vi "ConstructLabVIEWItem.vi"(8 "error in (no error)":errorcluster, 9 "Path":path, 10 "Qualified name":string, 11 "CLabVIEWItem in":refnum<class "CLabVIEWItem.lvclass">) -> (0 "error out":errorcluster, 3 "CLabVIEWItem out":refnum<class "CLabVIEWItem.lvclass">)   [LabVIEW 2020, in "LabVIEWItem.lvlib" / "CLabVIEWItem.lvclass"]
uses:
  CLabVIEWItem.lvclass
  CLabVIEWItem.lvclass/CLabVIEWItem.ctl
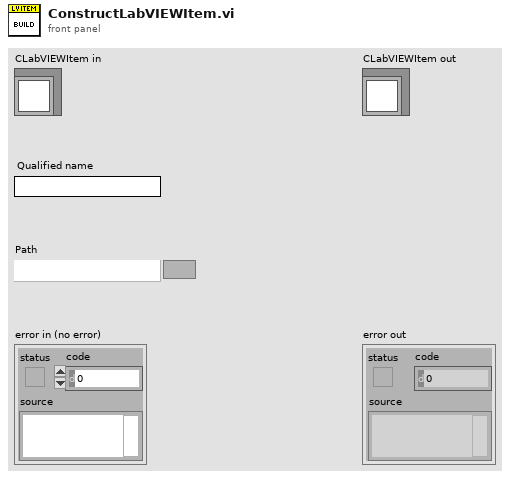
[diagram p1: front panel]
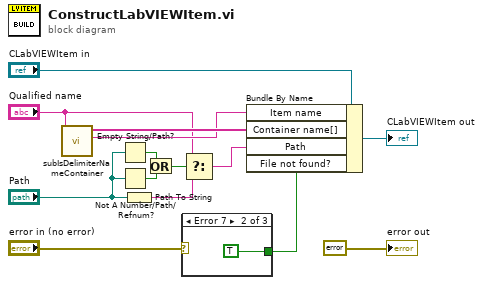
[diagram p0: block diagram]
diagram:
  n1 = call "subIsDelimiterNameContainer.vi"("delimited name"="Qualified name") -> ("item name"=w2:string, "container name[]"=w14:string[])  [unwired: 8 in, 1 out]
  n2 = Empty String/Path?(string/path="Path") -> (empty?=w12:bool)
  n3 = Not A Number/Path/Refnum?(number/path/refnum="Path") -> (NaN/Path/Refnum?=w11:bool)
  n4 = Path To String(path="Path") -> (string=w9:string)
  n5 = Or(x=w12, y=w11) -> (x .or. y?=w10:bool)
  n6 = case shown="Error 7" "error in (no error)" {
    tunnel: [_ TRUE _] -> w6
    frame No Error {
    }
    frame Error {
    }
    frame Default {
    }
  }
  n7 = Select(t="Qualified name", s=w10, f=w9) -> (s? t:f=w7:string)
  n8 = Bundle By Name(cluster="CLabVIEWItem in", "Item name"=w2, "Container name[]"=w14, "Path"=w7, "File not found?"=w6) -> (→"CLabVIEWItem out":refnum<class "CLabVIEWItem.lvclass">)
  "error out" <- errorcluster {"status"=FALSE, "code"=0, "source"=""} ("error out")
